vi "CameraSetParams.vi"(8 "error in (no error)":errorcluster, 10 "settings":T2={"exposure"=0.0, "external"=FALSE, "roi"={"left"=0, "top"=0, "right"=0, "bottom"=0}, "frames"=0, "bin_x"=1, "bin_y"=1}, 11 "AndorSDK2 in":refnum<class "Andor2.lvclass">) -> (0 "error out":errorcluster, 1 "roi_out":T1, 2 "attributes":variant[](array[variant]), 3 "AndorSDK2 out":refnum<class "Andor2.lvclass">)   [LabVIEW 2010, in "Andor2.lvclass"]
uses:
  Andor2.lvclass
  subvis/ExposureSettings.ctl
  subvis/ROI_rect.ctl
  <userlib>/Andor/atmcd32d.llb/AcquisitionMode_mode typedef.ctl
  <userlib>/Andor/atmcd32d.llb/ReadMode_mode typedef.ctl
  Andor2.lvclass/Andor2.ctl
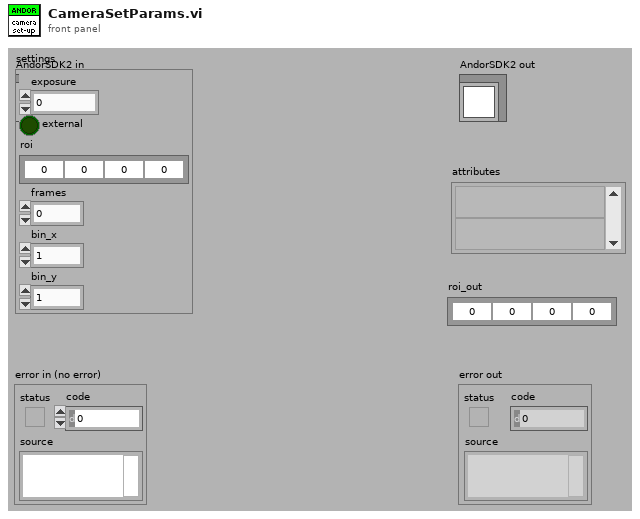
[diagram p1: front panel]
types:
  T1 = typedef "ROI_rect.ctl" = cluster{"left":i32, "top":i32, "right":i32, "bottom":i32}
  T2 = typedef "ExposureSettings.ctl" = cluster{"exposure":dbl, "external":bool, "roi":T1, "frames":i32, "bin_x":u8, "bin_y":u8}
  T3 = typedef "ReadMode_mode typedef.ctl" = enum16{"Full Vertical Binning", "Multi-Track", "Random-Track", "Single-Track", "Image"}
  T4 = typedef "AcquisitionMode_mode typedef.ctl" = enum16{"Reserved (0)", "Single Scan", "Accumulate", "Kinetics", "Fast Kinetics", "Run Till Abort", "Reserved (6)", "Reserved (7)", "Reserved (8)", "Time Delayed Integration"}
  T5 = cluster{"AD chan":i32, "HS index":i32, "HS speed":sgl, "VS index":i32, "VS speed":sgl}
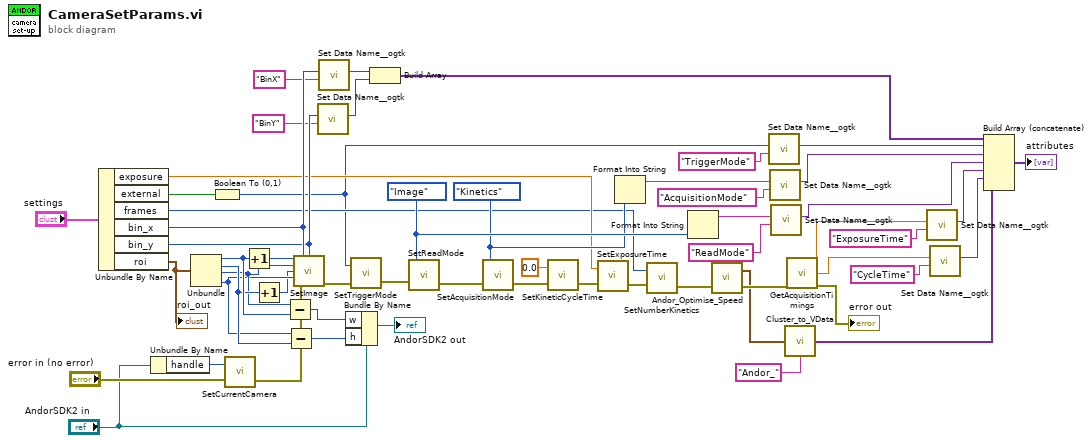
[diagram p0: block diagram]
diagram:
  w50 = ReadMode_mode_typedef."Image" ("mode")
  w49 = AcquisitionMode_mode_typedef."Kinetics" ("mode")
  n1 = Unbundle By Name("settings") -> ("exposure"=w14:dbl, "external"=w55:bool, "frames"=w12:i32, "bin_x"=w38:u8, "bin_y"=w37:u8, "roi"=w26:T1)
  "roi_out" <- w26
  n2 = Unbundle By Name("AndorSDK2 in") -> ("handle"=w52:i32)
  n3 = Unbundle(w26) -> ("left"=w30:i32, "top"=w27:i32, "right"=w24:i32, "bottom"=w23:i32)
  n4 = Boolean To (0,1)(Boolean=w55) -> (0, 1=w5:i16)
  n5 = call <userlib>:"SetCurrentCamera.vi"("error in (no error)"="error in (no error)", "cameraHandle"=w52) -> ("error out"=w54:errorcluster)  [unwired: 1 out]
  n6 = Increment(x=w30) -> (x+1=w25:i32)
  n7 = Increment(x=w27) -> (x+1=w22:i32)
  n8 = Subtract(x=w24, y=w30) -> (x-y=w29:i32)
  n9 = Subtract(x=w23, y=w27) -> (x-y=w28:i32)
  n10 = call <userlib>:"SetImage.vi"("hstart"=w25, "hbin"=w38, "vbin"=w37, "hend"=w24, "vstart"=w22, "vend"=w23, "error in (no error)"=w54) -> ("error out"=w9:errorcluster)  [unwired: 7 in, 1 out]
  n11 = call <userlib>:"Set Data Name__ogtk.vi"("Data Name"="BinY", "Data"=w37) -> ("Renamed Data"=w33:variant)  [unwired: 8 in, 1 out]
  n12 = call <userlib>:"Set Data Name__ogtk.vi"("Data Name"="BinX", "Data"=w38) -> ("Renamed Data"=w34:variant)  [unwired: 8 in, 1 out]
  n13 = Bundle By Name(cluster="AndorSDK2 in", "w"=w29, "h"=w28) -> (→"AndorSDK2 out":refnum<class "Andor2.lvclass">)
  n14 = call <userlib>:"SetTriggerMode.vi"("error in (no error)"=w9, "mode"=w5) -> ("error out"=w8:errorcluster)  [unwired: 1 out]
  n15 = Build Array(w34, w33) -> (w10:variant[])
  n16 = call <userlib>:"SetReadMode.vi"("error in (no error)"=w8, "mode"=w50) -> ("error out"=w17:errorcluster)  [unwired: 1 out]
  n17 = call <userlib>:"SetAcquisitionMode.vi"("error in (no error)"=w17, "mode"=w49) -> ("error out"=w16:errorcluster)  [unwired: 1 out]
  n18 = call <userlib>:"SetKineticCycleTime.vi"("error in (no error)"=w16, "time"=sgl 0.0) -> ("error out"=w15:errorcluster)  [unwired: 1 out]
  n19 = call <userlib>:"SetExposureTime.vi"("error in (no error)"=w15, "time"=w14) -> ("error out"=w13:errorcluster)  [unwired: 1 out]
  n20 = Format Into String(w49) -> (resulting string=w47:string)  [unwired: 3 in, 1 out]
  n21 = call <userlib>:"SetNumberKinetics.vi"("error in (no error)"=w13, "number"=w12) -> ("error out"=w11:errorcluster)  [unwired: 1 out]
  n22 = Format Into String(w50) -> (resulting string=w45:string)  [unwired: 3 in, 1 out]
  n23 = call <userlib>:"Andor_Optimise_Speed.vi"("error in"=w11) -> ("error out"=w4:errorcluster, "params"=w3:T5)  [unwired: 1 in]
  n24 = call <userlib>:"Set Data Name__ogtk.vi"("Data Name"="TriggerMode", "Data"=w5) -> ("Renamed Data"=w7:variant)  [unwired: 8 in, 1 out]
  n25 = call <userlib>:"Set Data Name__ogtk.vi"("Data Name"="AcquisitionMode", "Data"=w47) -> ("Renamed Data"=w39:variant)  [unwired: 8 in, 1 out]
  n26 = call <userlib>:"Set Data Name__ogtk.vi"("Data Name"="ReadMode", "Data"=w45) -> ("Renamed Data"=w40:variant)  [unwired: 8 in, 1 out]
  n27 = call "Cluster_to_VData.vi"("cluster"=w3, "prefix"="Andor_") -> ("vdata"=w1:variant[])
  n28 = call <userlib>:"GetAcquisitionTimings.vi"("error in (no error)"=w4) -> ("exposure"=w43:sgl, "kinetic"=w19:sgl, "error out"=→"error out":errorcluster)  [unwired: 10 in, 2 out]
  n29 = call <userlib>:"Set Data Name__ogtk.vi"("Data Name"="ExposureTime", "Data"=w43) -> ("Renamed Data"=w41:variant)  [unwired: 8 in, 1 out]
  n30 = call <userlib>:"Set Data Name__ogtk.vi"("Data Name"="CycleTime", "Data"=w19) -> ("Renamed Data"=w18:variant)  [unwired: 8 in, 1 out]
  n31 = Build Array (concatenate)(w10, w7, w39, w40, w41, w18, w1) -> (→"attributes":variant[])
